vi "Update.vi"(8 "error in (no error)":errorcluster, 10 "Engine in":refnum<class "Engine.lvclass">, 11 "Snake in":refnum<class "SnakeDemo.lvclass">) -> (0 "error out":errorcluster, 2 "Engine out":refnum<class "Engine.lvclass">, 3 "Snake out":refnum<class "SnakeDemo.lvclass">)   [LabVIEW 2019, in "RT_Game.lvlib" / "SnakeDemo.lvclass"]
uses:
  SnakeDemo.lvclass
  C:/Users/FreshBob/Dropbox/VIs/myRIO_GameConsole/RT/RT_Game/Game/Game.lvclass
  C:/Users/FreshBob/Dropbox/VIs/myRIO_GameConsole/RT/RT_Game/SnakeGame/SnakeGame.lvclass
  Engine/Engine.lvclass
  Game/Game.lvclass/Game.ctl
  SnakeGame/SnakeGame.lvclass/SnakeGame.ctl
  AttractScreen/AttractScreen.lvclass
  Engine/Engine.lvclass/Engine.ctl
  SnakeGame/Write Winner_.vi
  Engine/Write NextGame.vi
  Engine/Write SwitchGame_.vi
  Game/Read State.vi
  SnakeGame/SnakeGame.lvclass
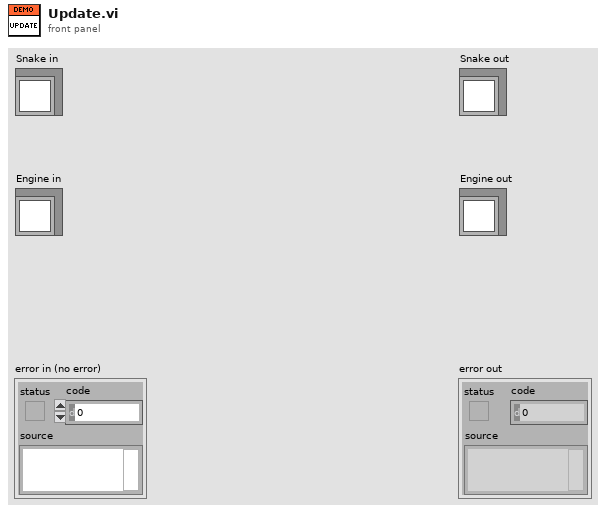
[diagram p1: front panel]
types:
  T1 = typedef "RT_Game.lvlib/Game.lvclass/States.ctl" = enum16{"Init", "Restart", "Menu", "Game", "Resume", "ToggleSingleplayer", "LoadNextGame", "ExitToMenu", "NewHighscore", "GameOver", "SlideOut", "FadeToMenu", "StartFadeToMenu"}
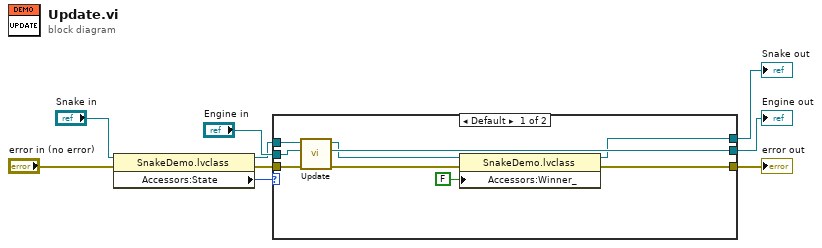
[diagram p0: block diagram]
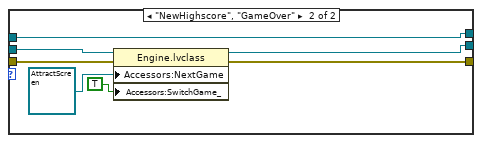
[diagram p2: hidden frame]
diagram:
  n1 = property class="SnakeDemo.lvclass"(reference="Snake in", error in="error in (no error)") -> (reference out=w2:refnum<class "SnakeDemo.lvclass">, error out=w6:errorcluster, "Accessors:State"=w3:T1)
  n2 = case shown="Default" w3 {
    tunnel: w6 -> [w18 w25]
    tunnel: [w13 w24] -> w5
    tunnel: "Engine in" -> [w15 w23]
    tunnel: [w14 w22] -> w4
    tunnel: w2 -> [w16 w19]
    tunnel: [w11 w19] -> w1
    frame Default {
      n3 = call-parent "Update.vi"("error in (no error)"=w18, "Engine in"=w15, "Snake in"=w16) -> ("error out"=w17:errorcluster, "Engine out"=w14:refnum<class "Engine.lvclass">, "Snake out"=w12:refnum<class "SnakeDemo.lvclass">)  [unwired: 6 in]
      n4 = property class="SnakeDemo.lvclass"(reference=w12, error in=w17, "Accessors:Winner_"=FALSE ("Winner_")) -> (reference out=w11:refnum<class "SnakeDemo.lvclass">, error out=w13:errorcluster)
    }
    frame "NewHighscore", "GameOver" {
      n5 = property class="Engine.lvclass"(reference=w23, error in=w25, "Accessors:NextGame"=refnum<class "AttractScreen.lvclass"> refnum ("RT_Game.lvlib:AttractScreen.lvclass"), "Accessors:SwitchGame_"=TRUE ("SwitchGame_")) -> (reference out=w22:refnum<class "Engine.lvclass">, error out=w24:errorcluster)
    }
  }
  "error out" <- w5
  "Engine out" <- w4
  "Snake out" <- w1
